vi "Begin.vi"(8 "error in":errorcluster) -> (0 "error out":errorcluster)   [LabVIEW 2016]
doc: "Called before other user functions, this VI is expected to open initial I/O refnums, load in file data, and do all program initialization. Notice that the <B>error out</B> terminal is simply used for data flow. Wiring it to other structures or subVIs ensures that this VI runs first."
uses:
  <vilib>/Rock Robotics/WPI/DriverStation/WPI_DriverStationRobotMode2.ctl
  <vilib>/Rock Robotics/WPI/Joystick/WPI_JoystickDeviceEnum.ctl
  <vilib>/Rock Robotics/SystemInterfaces/AI/FPGA_AIChannel.ctl
  <vilib>/Rock Robotics/SystemInterfaces/DIO/FPGA_DIOChannel.ctl
  <vilib>/Rock Robotics/SystemInterfaces/DIO/FPGA_DIOPWMChannel.ctl
  <vilib>/Rock Robotics/WPI/Solenoid/WPI_SolenoidChannel.ctl
  <vilib>/Rock Robotics/WPI/ThirdParty/CanMotor/TalonSRX/WPI_CANTalonSRX_APIControlMode.ctl
  <vilib>/Rock Robotics/WPI/ThirdParty/CanMotor/TalonSRX/WPI_CANTalonSRX_BrakeOverride.ctl
  <vilib>/Rock Robotics/SystemInterfaces/AI/FPGA_AIGyroChannel.ctl
  <vilib>/Rock Robotics/Network Tables/NT Write String Array.vi
  <vilib>/Rock Robotics/WPI/Ultrasonic/WPI_SonarMB1010AnalogOpen.vi
  <vilib>/Rock Robotics/WPI/Ultrasonic/WPI_SonarMB1010AnalogRefNum Registry Set.vi
  <vilib>/Rock Robotics/WPI/Switch/WPI_SwitchOpenLimit.vi
  <vilib>/Rock Robotics/WPI/Solenoid/WPI_SolenoidOpenSingle.vi
  Robot Global Data.vi
  2039lib.lvlib
panel:
  in  "Robot Mode":T1
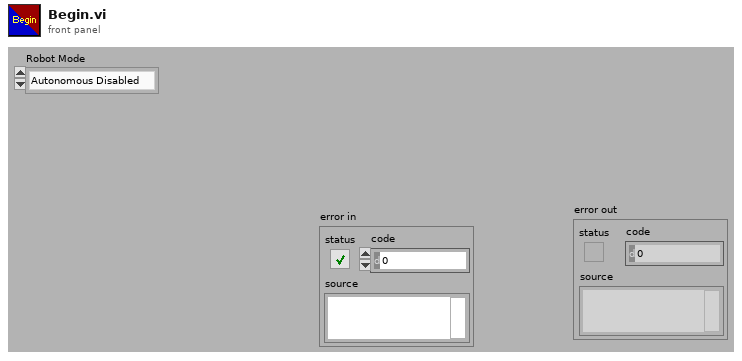
[diagram p1: front panel]
types:
  T1 = typedef "WPI_DriverStationRobotMode2.ctl" = enum16{"Autonomous Disabled", "Autonomous Enabled", "Teleop Disabled", "Teleop Enabled", "Disconnected", "Finish", "Test Disabled", "Test Enabled", "Emergency Stopped"}
  T2 = typedef "FPGA_AIGyroChannel.ctl" = enum8{"AI 0", "AI 1", "Invalid"}
  T3 = typedef "WPI_CANTalonSRX_BrakeOverride.ctl" = enum8{"No Override", "Override to Coast", "Override to Brake"}
  T4 = typedef "WPI_CANTalonSRX_APIControlMode.ctl" = enum8{"Percent VBus", "Speed", "Position", "Slave", "Unchanged / Invalid", "Voltage Compensation", "Current", "Motion Profile", "Motion Magic"}
  T5 = typedef "WPI_SolenoidChannel.ctl" = enum8{"Solenoid 0", "Solenoid 1", "Solenoid 2", "Solenoid 3", "Solenoid 4", "Solenoid 5", "Solenoid 6", "Solenoid 7", "Invalid"}
  T6 = typedef "FPGA_DIOPWMChannel.ctl" = enum8{"PWM 0", "PWM 1", "PWM 2", "PWM 3", "PWM 4", "PWM 5", "PWM 6", "PWM 7", "PWM 8", "PWM 9", "PWM MXP 0", "PWM MXP 1", "PWM MXP 2", "PWM MXP 3", "PWM MXP 4", "PWM MXP 5", "PWM MXP 6", "PWM MXP 7", "PWM MXP 8", "PWM MXP 9", "Invalid"}
  T7 = typedef "FPGA_DIOChannel.ctl" = enum8{"DIO 0", "DIO 1", "DIO 2", "DIO 3", "DIO 4", "DIO 5", "DIO 6", "DIO 7", "DIO 8", "DIO 9", "DIO MXP 0", "DIO MXP 1", "DIO MXP 2", "DIO MXP 3", "DIO MXP 4", "DIO MXP 5", "DIO MXP 6", "DIO MXP 7", "DIO MXP 8", "DIO MXP 9", "DIO MXP 10", "DIO MXP 11", "DIO MXP 12", "DIO MXP 13", "DIO MXP 14", "DIO MXP 15", "SPI Port CS1", "SPI Port CS2", "SPI Port CS3", "SPI Port MISO", "SPI Port MOSI", "Invalid"}
  T8 = typedef "WPI_JoystickDeviceEnum.ctl" = enum16{"USB 0", "USB 1", "USB 2", "USB 3", "USB 4", "USB 5"}
  T9 = typedef "FPGA_AIChannel.ctl" = enum8{"AI 0", "AI 1", "AI 2", "AI 3", "AI MXP 0", "AI MXP 1", "AI MXP 2", "AI MXP 3", "Invalid"}
  T10 = typedef "WPI_SonarMB1010AnalogDeviceRef.ctl" = cluster{"AIDeviceRef":T11, "Scaling factor (V/in)":dbl, "Average Bits":u8}
  T11 = typedef "WPI_AnalogChannelDevRef.ctl" = cluster{"DevStatus":errorcluster, "Analog Channel":T9}
  T12 = typedef "WPI_MotorControlDeviceRef.ctl" = cluster{"DeviceStatus":errorcluster, "Type":T13, "PWM":cluster{"PWM Channel":T6, "DeadBand":T14}, "CAN":cluster{"Device Number":u8, "SetOutput VI Ref":variant, "GetOutput VI Ref":variant, "Enable VI Ref":variant, "Disable VI Ref":variant, "Data":variant}, "Invert":bool}
  T13 = typedef "WPI_MotorControlType.ctl" = enum16{"PWM", "CAN"}
  T14 = typedef "WPI_PWMDeadband.ctl" = cluster{"Name":string, "maxPositivePwm":i32, "minPositivePwm":i32, "centerPwm":i32, "maxNegativePwm":i32, "minNegativePwm":i32, "angularRange":u16}
  T15 = typedef "WPI_JoystickDevRef.ctl" = cluster{"Device":T8}
  T16 = typedef "WPI_SwitchDevRef.ctl" = cluster{"DevStatus":errorcluster, "DIO Channel":T7, "CntIndex":T17, "Normally Closed":bool}
  T17 = typedef "FPGA_CounterCtrSystemIndex.ctl" = enum8{"Ctr 0", "Ctr 1", "Ctr 2", "Ctr 3", "Ctr 4", "Ctr 5", "Ctr 6", "Ctr 7", "Invalid"}
  T18 = typedef "WPI_GyroDevRef.ctl" = cluster{"DevStatus":errorcluster, "Analog Channel":T9, "Offset":dbl, "Gain (VoltsPerDegree/Second)":dbl, "Gyro Type":enum16{"Analog", "XRS450"}, "Handle":i32, "SPI Bus":T19, "Device Found":bool, "Sample Rate":dbl, "Calibrate On Open":bool}
  T19 = typedef "spi_bus.ctl" = enum16{"SPI On-Board, CS0", "SPI On-Board, CS1", "SPI On-Board, CS2", "SPI On-Board, CS3", "SPI MXP", "Invalid"}
  T20 = typedef "WPI_AccelerometerDevRef.ctl" = cluster{"DevStatus":errorcluster, "Scaling":T21, "Analog Channels":T22, "I2C Bus":T23, "SPI Bus":T19, "Accel Range":T24, "ADXL Axes":T25, "Handle":i32, "Device Address":u8, "Accel Type":enum16{"Analog", "ADXL345 I2C", "ADXL345 SPI", "Internal", "ADXL362 SPI"}}
  T21 = typedef "WPI_AccelerometerScaling.ctl" = cluster{"Gain (VoltsPerG)":dbl, "Center Voltage":dbl}
  T22 = typedef "WPI_AccelerometerAnalogChannels.ctl" = cluster{"X-Axis":T9, "Y-Axis":T9, "Z-Axis":T9}
  T23 = typedef "i2c_bus.ctl" = enum16{"I2C On-Board", "I2C MXP", "Invalid"}
  T24 = typedef "ADXL345 Range.ctl" = u8
  T25 = typedef "WPI_AccelerometerADXL345 Axes.ctl" = cluster{"X-Axis":bool, "Y-Axis":bool, "Z-Axis":bool}
  T26 = cluster{"GyroDevRef":T18, "AccelerometerDevRef":T20}
  T27 = typedef "WPI_ServoDeviceRef.ctl" = cluster{"DeviceStatus":errorcluster, "PWM Channel":T6, "DeadBand":T14}
  T28 = typedef "WPI_DigitalInputDevRef.ctl" = cluster{"DevStatus":errorcluster, "DIO Channel":T7}
  T29 = typedef "WPI_SolenoidDevRef.ctl" = cluster{"DevStatus":errorcluster, "Pneumatics Control Module":u8, "Forward Solenoid Channel":T5, "Reverse Solenoid Channel":T5}
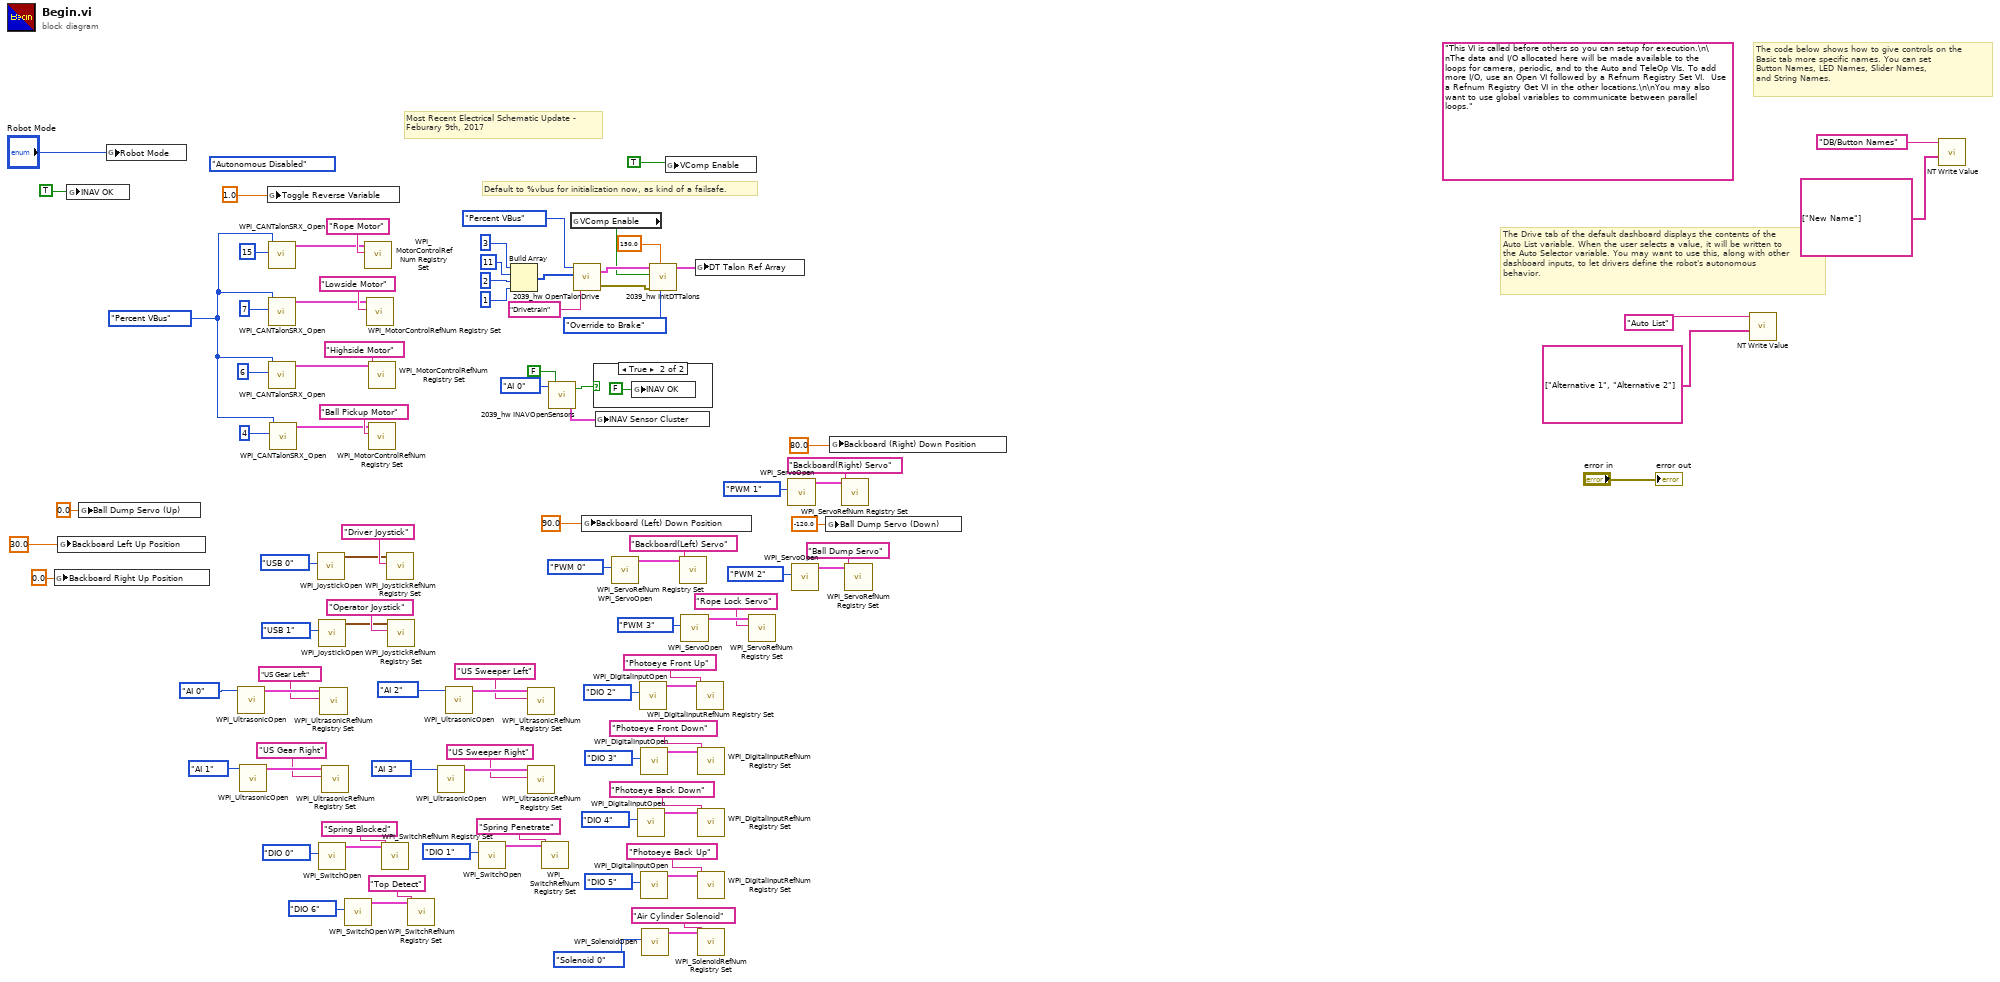
[diagram p0: block diagram]
diagram:
  w40 = WPI_CANTalonSRX_APIControlMode."Percent VBus" ("Control Mode")
  (unwired) WPI_DriverStationRobotMode2."Autonomous Disabled" ("Robot Mode")
  (unwired) "This VI is called before others so you can setup for execution.\n\nThe data and I/O allocated here will be made available to the loops for camera, periodic, and to the Auto and TeleOp VIs. To add more I/O, use an Open VI followed by a Refnum Registry Set VI.  Use a Refnum Registry Get VI in the other locations.\n\nYou may also want to use global variables to communicate between parallel loops."
  # "Default to %vbus for initialization now, as kind of a failsafe."
  # "Most Recent Electrical Schematic Update -\nFeburary 9th, 2017"
  # "The Drive tab of the default dashboard displays the contents of the\nAuto List variable. When the user selects a value, it will be written to\nthe Auto Selector variable. You may want to use this, along with other\ndashboard inputs, to let drivers define the robot's autonomous\nbehavior."
  # "The code below shows how to give controls on the\nBasic tab more specific names. You can set\nButton Names, LED Names, Slider Names,\nand String Names."
  n1 = global write "Robot Global Data.vi" "Backboard Right Up Position"(0.0 ("Backboard Right Up Position")) -> ()
  n2 = global write "Robot Global Data.vi" "Backboard Left Up Position"(30.0 ("Backboard Left Up Position")) -> ()
  n3 = global write "Robot Global Data.vi" "INAV OK"(TRUE) -> ()
  n4 = global write "Robot Global Data.vi" "Ball Dump Servo (Up)"(0.0 ("Ball Dump Servo (Up)")) -> ()
  n5 = global write "Robot Global Data.vi" "Robot Mode"("Robot Mode") -> ()
  n6 = call-poly <vilib>:"WPI_UltrasonicOpen.vi"("Analog Channel"=FPGA_AIChannel."AI 0") -> ("SonarMB1010AnalogDevRef"=w90:T10)  [unwired: 9 in, 1 out]
  n7 = call-poly <vilib>:"WPI_UltrasonicOpen.vi"("Analog Channel"=FPGA_AIChannel."AI 1") -> ("SonarMB1010AnalogDevRef"=w87:T10)  [unwired: 9 in, 1 out]
  n8 = global write "Robot Global Data.vi" "Toggle Reverse Variable"(1.0 ("Toggle Reverse Variable")) -> ()
  n9 = call <vilib>:"WPI_CANTalonSRX_Open.vi"("Device Number"=15, "Control Mode"=w40) -> ("CAN Talon SRX Ref"=w34:T12)  [unwired: 8 in, 1 out]
  n10 = call <vilib>:"WPI_CANTalonSRX_Open.vi"("Device Number"=7, "Control Mode"=w40) -> ("CAN Talon SRX Ref"=w33:T12)  [unwired: 8 in, 1 out]
  n11 = call <vilib>:"WPI_CANTalonSRX_Open.vi"("Device Number"=6, "Control Mode"=w40) -> ("CAN Talon SRX Ref"=w32:T12)  [unwired: 8 in, 1 out]
  n12 = call <vilib>:"WPI_CANTalonSRX_Open.vi"("Device Number"=4, "Control Mode"=w40) -> ("CAN Talon SRX Ref"=w31:T12)  [unwired: 8 in, 1 out]
  n13 = call <vilib>:"WPI_JoystickOpen.vi"("JoystickDevice"=WPI_JoystickDeviceEnum."USB 0") -> ("JoystickDevRef"=w98:T15)  [unwired: 10 in]
  n14 = call <vilib>:"WPI_JoystickOpen.vi"("JoystickDevice"=WPI_JoystickDeviceEnum."USB 1") -> ("JoystickDevRef"=w78:T15)  [unwired: 10 in]
  n15 = call-poly <vilib>:"WPI_SwitchOpen.vi"("DIO Channel"=FPGA_DIOChannel."DIO 0") -> ("SwitchDevRef"=w76:T16)  [unwired: 9 in, 1 out]
  n16 = call-poly <vilib>:"WPI_UltrasonicRefNum Registry Set.vi"("refnum name"="US Gear Left", "SonarMB1010AnalogDevRef"=w90) -> ()  [unwired: 8 in, 2 out]
  n17 = call-poly <vilib>:"WPI_UltrasonicRefNum Registry Set.vi"("refnum name"="US Gear Right", "SonarMB1010AnalogDevRef"=w87) -> ()  [unwired: 8 in, 2 out]
  n18 = call-poly <vilib>:"WPI_SwitchOpen.vi"("DIO Channel"=FPGA_DIOChannel."DIO 6") -> ("SwitchDevRef"=w53:T16)  [unwired: 9 in, 1 out]
  n19 = call <vilib>:"WPI_MotorControlRefNum Registry Set.vi"("refnum name"="Rope Motor", "MotorControlDevRef"=w34) -> ()  [unwired: 8 in, 2 out]
  n20 = call <vilib>:"WPI_MotorControlRefNum Registry Set.vi"("refnum name"="Lowside Motor", "MotorControlDevRef"=w33) -> ()  [unwired: 8 in, 2 out]
  n21 = call <vilib>:"WPI_MotorControlRefNum Registry Set.vi"("refnum name"="Highside Motor", "MotorControlDevRef"=w32) -> ()  [unwired: 8 in, 2 out]
  n22 = call <vilib>:"WPI_MotorControlRefNum Registry Set.vi"("refnum name"="Ball Pickup Motor", "MotorControlDevRef"=w31) -> ()  [unwired: 8 in, 2 out]
  n23 = call <vilib>:"WPI_SwitchRefNum Registry Set.vi"("refnum name"="Spring Blocked", "SwitchDevRef"=w76) -> ()  [unwired: 8 in, 2 out]
  n24 = call <vilib>:"WPI_JoystickRefNum Registry Set.vi"("refnum name"="Driver Joystick", "JoystickDevRef"=w98) -> ()  [unwired: 8 in, 2 out]
  n25 = call <vilib>:"WPI_JoystickRefNum Registry Set.vi"("refnum name"="Operator Joystick", "JoystickDevRef"=w78) -> ()  [unwired: 8 in, 2 out]
  n26 = call <vilib>:"WPI_SwitchRefNum Registry Set.vi"("refnum name"="Top Detect", "SwitchDevRef"=w53) -> ()  [unwired: 8 in, 2 out]
  n27 = call-poly <vilib>:"WPI_UltrasonicOpen.vi"("Analog Channel"=FPGA_AIChannel."AI 3") -> ("SonarMB1010AnalogDevRef"=w81:T10)  [unwired: 9 in, 1 out]
  n28 = call-poly <vilib>:"WPI_UltrasonicOpen.vi"("Analog Channel"=FPGA_AIChannel."AI 2") -> ("SonarMB1010AnalogDevRef"=w84:T10)  [unwired: 9 in, 1 out]
  n29 = call-poly <vilib>:"WPI_SwitchOpen.vi"("DIO Channel"=FPGA_DIOChannel."DIO 1") -> ("SwitchDevRef"=w73:T16)  [unwired: 9 in, 1 out]
  n30 = Build Array(u8 3 ("Device Number"), u8 11 ("Device Number"), u8 2 ("Device Number"), u8 1 ("Device Number")) -> (w24:u8[])
  n31 = call-poly <vilib>:"WPI_UltrasonicRefNum Registry Set.vi"("refnum name"="US Sweeper Left", "SonarMB1010AnalogDevRef"=w84) -> ()  [unwired: 8 in, 2 out]
  n32 = call-poly <vilib>:"WPI_UltrasonicRefNum Registry Set.vi"("refnum name"="US Sweeper Right", "SonarMB1010AnalogDevRef"=w81) -> ()  [unwired: 8 in, 2 out]
  n33 = call <vilib>:"WPI_SwitchRefNum Registry Set.vi"("refnum name"="Spring Penetrate", "SwitchDevRef"=w73) -> ()  [unwired: 8 in, 2 out]
  n34 = call "2039_hw INAVOpenSensors.vi"("Use External Accel"=FALSE, "Gyroscope Analog Channel"=FPGA_AIGyroChannel."AI 0") -> ("INAV Sensor Cluster"=w13:T26, "INAV Not OK"=w12:bool)  [unwired: 1 in]
  n35 = global read "Robot Global Data.vi" "VComp Enable"() -> (w19:bool)
  n36 = call "2039_hw OpenTalonDrive.vi"("refnum name"="Drivetrain", "CAN IDs"=w24, "Control Mode"=WPI_CANTalonSRX_APIControlMode."Percent VBus") -> ("error out"=w20:errorcluster, "Drivetrain Talon SRX Ref Array"=w21:T12[])  [unwired: 1 in]
  n37 = global write "Robot Global Data.vi" "Backboard (Left) Down Position"(90.0 ("Toggle Reverse Variable")) -> ()
  n38 = case shown="True" w12 {
    frame False {
    }
    frame True {
      n39 = global write "Robot Global Data.vi" "INAV OK"(FALSE) -> ()
    }
  }
  n40 = global write "Robot Global Data.vi" "INAV Sensor Cluster"(w13) -> ()
  n41 = call <vilib>:"WPI_ServoOpen.vi"("PWM Channel"=FPGA_DIOPWMChannel."PWM 0") -> ("ServoDeviceRef"=w1:T27)  [unwired: 9 in, 1 out]
  n42 = call <vilib>:"WPI_DigitalInputOpen.vi"("DIO Channel"=FPGA_DIOChannel."DIO 4") -> ("DigitalInputDevRef"=w47:T28)  [unwired: 9 in, 1 out]
  n43 = call <vilib>:"WPI_DigitalInputOpen.vi"("DIO Channel"=FPGA_DIOChannel."DIO 2") -> ("DigitalInputDevRef"=w63:T28)  [unwired: 9 in, 1 out]
  n44 = call <vilib>:"WPI_DigitalInputOpen.vi"("DIO Channel"=FPGA_DIOChannel."DIO 3") -> ("DigitalInputDevRef"=w60:T28)  [unwired: 9 in, 1 out]
  n45 = call <vilib>:"WPI_DigitalInputOpen.vi"("DIO Channel"=FPGA_DIOChannel."DIO 5") -> ("DigitalInputDevRef"=w55:T28)  [unwired: 9 in, 1 out]
  n46 = call-poly <vilib>:"WPI_SolenoidOpen.vi"("Solenoid Channel"=WPI_SolenoidChannel."Solenoid 0") -> ("SolenoidDevRef"=w46:T29)  [unwired: 9 in, 1 out]
  n47 = call "2039_hw InitDTTalons.vi"("Brake / Coast Mode"=WPI_CANTalonSRX_BrakeOverride."Override to Brake", "Ramp Rate (Percent/s)"=150.0, "error in (no error)"=w20, "Enable VComp"=w19, "DT Talon Ref Array"=w21) -> ("DT Talon Ref Array"=w10:T12[])  [unwired: 5 in, 1 out]
  n48 = global write "Robot Global Data.vi" "VComp Enable"(TRUE) -> ()
  n49 = call <vilib>:"WPI_ServoRefNum Registry Set.vi"("refnum name"="Backboard(Left) Servo", "ServoDeviceRef"=w1) -> ()  [unwired: 8 in, 2 out]
  n50 = call <vilib>:"WPI_ServoOpen.vi"("PWM Channel"=FPGA_DIOPWMChannel."PWM 3") -> ("ServoDeviceRef"=w49:T27)  [unwired: 9 in, 1 out]
  n51 = global write "Robot Global Data.vi" "DT Talon Ref Array"(w10) -> ()
  n52 = call <vilib>:"WPI_DigitalInputRefNum Registry Set.vi"("refnum name"="Photoeye Front Up", "DigitalInputDevRef"=w63) -> ()  [unwired: 8 in, 2 out]
  n53 = call <vilib>:"WPI_DigitalInputRefNum Registry Set.vi"("refnum name"="Photoeye Front Down", "DigitalInputDevRef"=w60) -> ()  [unwired: 8 in, 2 out]
  n54 = call <vilib>:"WPI_DigitalInputRefNum Registry Set.vi"("refnum name"="Photoeye Back Down", "DigitalInputDevRef"=w47) -> ()  [unwired: 8 in, 2 out]
  n55 = call <vilib>:"WPI_DigitalInputRefNum Registry Set.vi"("refnum name"="Photoeye Back Up", "DigitalInputDevRef"=w55) -> ()  [unwired: 8 in, 2 out]
  n56 = call <vilib>:"WPI_SolenoidRefNum Registry Set.vi"("refnum name"="Air Cylinder Solenoid", "SolenoidDevRef"=w46) -> ()  [unwired: 8 in, 2 out]
  n57 = call <vilib>:"WPI_ServoRefNum Registry Set.vi"("refnum name"="Rope Lock Servo", "ServoDeviceRef"=w49) -> ()  [unwired: 8 in, 2 out]
  n58 = call <vilib>:"WPI_ServoOpen.vi"("PWM Channel"=FPGA_DIOPWMChannel."PWM 1") -> ("ServoDeviceRef"=w2:T27)  [unwired: 9 in, 1 out]
  n59 = call <vilib>:"WPI_ServoOpen.vi"("PWM Channel"=FPGA_DIOPWMChannel."PWM 2") -> ("ServoDeviceRef"=w3:T27)  [unwired: 9 in, 1 out]
  n60 = global write "Robot Global Data.vi" "Ball Dump Servo (Down)"(-120.0 ("Ball Dump Servo (Down)")) -> ()
  n61 = global write "Robot Global Data.vi" "Backboard (Right) Down Position"(80.0 ("Toggle Reverse Variable")) -> ()
  n62 = call <vilib>:"WPI_ServoRefNum Registry Set.vi"("refnum name"="Backboard(Right) Servo", "ServoDeviceRef"=w2) -> ()  [unwired: 8 in, 2 out]
  n63 = call <vilib>:"WPI_ServoRefNum Registry Set.vi"("refnum name"="Ball Dump Servo", "ServoDeviceRef"=w3) -> ()  [unwired: 8 in, 2 out]
  n64 = call-poly <vilib>:"NT Write Value.vi"("String Array"=string[] ["Alternative 1", "Alternative 2"], "Name"="Auto List") -> ()  [unwired: 9 in, 1 out]
  n65 = call-poly <vilib>:"NT Write Value.vi"("String Array"=string[] ["New Name"], "Name"="DB/Button Names") -> ()  [unwired: 9 in, 1 out]
  "error out" <- "error in"
